vi "主程序.vi"() -> ()   [LabVIEW 2017, in "年前程序.lvlib"]
uses:
  <vilib>/Platform/TimedLoop/XDataNode/timing_clust.ctl
  <vilib>/Platform/TimedLoop/XDataNode/nitl_modes.ctl
  <vilib>/Platform/TimedLoop/XDataNode/wakeup.ctl
  <vilib>/myRIO/Common/Instrument Driver Framework/myRIO v1.0/UART/vis/myRIO v1.0 Close UART.vi
  <vilib>/FPGAPlugInAG/myRIO-1900/niLvFpga_Open_myRIO-1900.vi
  <vilib>/rvi/interface/common/dynamic/niFpgaDynamicAddResources.vi
  <vilib>/myRIO/Common/Instrument Driver Framework/Utilities/vis/FPGA Ref Manager.vi
  <vilib>/Utility/error.llb/Error Cluster From Error Code.vi
  <vilib>/myRIO/Common/Instrument Driver Framework/Utilities/vis/Ref Counter.vi
  <vilib>/FPGAPlugInAG/Dynamic/niLvFpga_Close_Dynamic.vi
  <vilib>/myRIO/Common/Instrument Driver Framework/myRIO v1.0/myRIO v1.0 Reset FPGA.vi
  <vilib>/myRIO/Common/Instrument Driver Framework/myRIO v1.0/IRQ/vis/myRIO v1.0 IRQ Info FGV.vi
  <vilib>/myRIO/Common/Instrument Driver Framework/myRIO v1.0/IRQ/vis/myRIO v1.0 Timer IRQ Info FGV.vi
  <vilib>/myRIO/Common/Instrument Driver Framework/myRIO v1.0/IRQ/vis/myRIO v1.0 ISR Agent.vi
  <vilib>/rvi/interface/nirviOpenFPGA/nirviOpenFPGA.xnode
  <vilib>/Platform/TimedLoop/XDataNode/XDataNode.xnode
  <vilib>/rvi/interface/nirviCloseFPGA/nirviCloseFPGA.xnode
  <vilib>/Platform/TimedLoop/XDataNode/XDNodeRunTimeDep.lvlib
  <vilib>/myRIO/Instrument Drivers/Utilities/Utilities.lvlib
panel:
  in  "最大速度":dbl
  in  "停止":bool
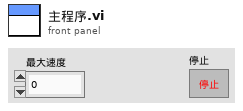
[diagram p1: front panel]
types:
  T1 = typedef "XDNodeRunTimeDep.lvlib/timing_clust.ctl" = cluster{"Expected End [f-1]":u64, "Actual End [f-1]":u64, "Finished Late? [f-1]":bool, "Expected End [i-1]":u64, "Actual End [i-1]":u64, "Finished Late? [i-1]":bool, "Expected Start [i]":u64, "Actual Start [i]":u64, "Expected Start [f]":u64, "Actual Start [f]":u64, "Source Name":string, "Structure Name":string, "Period":i64, "Deadline":i64, "Offset":i64, "Start":i64, "Priority":i32, "Timeout":i32, "Mode":T2, "Wakeup Reason":T3, "Error":errorcluster, "Source Type":string, "Secondary Source Type":string, "Global End Time":u64, "Global Start Time":u64, "Frame Duration":u64, "Iteration Duration":u64, "Assigned CPU":i32, "I/O Scan Engine Mode":u32}
  T2 = typedef "XDNodeRunTimeDep.lvlib/nitl_modes.ctl" = enum32{"No Change", "Process missed periods, maintain original phase", "Discard missed periods, maintain original phase", "Process missed periods, ignore original phase", "Discard missed periods, ignore original phase"}
  T3 = typedef "XDNodeRunTimeDep.lvlib/wakeup.ctl" = enum32{"Normal", "Aborted", "Asynchronous wakeup", "Timing source error", "Timed loop error", "Timeout"}
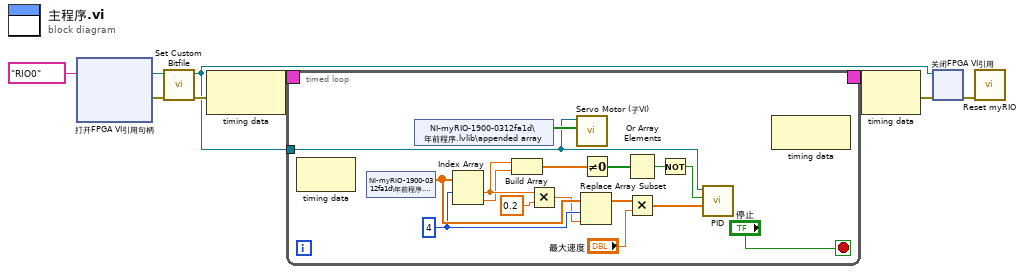
[diagram p0: block diagram]
diagram:
  n1 = xnode "打开FPGA VI引用句柄"("资源名称"=tag "RIO0") -> ("FPGA VI引用输出"=w5:refnum<k20>, "错误输出"=w4:errorcluster)  [unwired: 1 in]
  n2 = call <vilib>:"Set Custom Bitfile.vi"("error in (no error)"=w4, "Custom FPGA Reference In"=w5) -> ("error out"=w2:errorcluster, "Custom FPGA Reference Out"=w1:refnum<k20>)  [unwired: 8 in]
  n3 = node-c288(w2) -> (w9:T1)
  n4 = timed-loop {
    timing: w9 -> [_]
    timing-out: [_] -> w8
    tunnel: w1 -> [w21]
    stop <- "停止" stop-if-true
    w18 = 4 ("索引")
    n5 = node-c288() -> ()  [unwired: 1 in, 1 out]
    n6 = shared-variable "NI-myRIO-1900-0312fa1d\\年前程序.lvlib\\数组"() -> (w20:dbl[])  [unwired: 1 in, 1 out]
    n7 = shared-variable "NI-myRIO-1900-0312fa1d\\年前程序.lvlib\\appended array"() -> (w22:bool[])  [unwired: 1 in, 1 out]
    n8 = Index Array(array=w20, index #1=w18) -> (element #1=w15:dbl, element #2=w14:dbl)  [unwired: 1 in]
    n9 = Build Array(w15, w14) -> (w13:dbl[])
    n10 = Multiply(x=w15, y=0.2 ("x")) -> (x*y=w17:dbl)
    n11 = call "Servo Motor (子VI).vi"("Direction"=w22, "Custom FPGA Reference Out"=w21) -> ()  [unwired: 10 in]
    n12 = Replace Array Subset(array=w20, new element=w17, index=w18) -> (w19:dbl[])
    n13 = Not Equal To 0?(x=w13) -> (x != 0?=w12:bool[])
    n14 = Or Array Elements(Boolean array=w12) -> (logical OR=w11:bool)
    n15 = Multiply(x=w19, y="最大速度") -> (x*y=w23:dbl[])
    n16 = Not(x=w11) -> (.not. x?=w10:bool)
    n17 = call "PID.vi"("setpoint"=w23, "Relay"=w10, "Custom FPGA Reference Out"=w21) -> ()  [unwired: 9 in]
    n18 = node-c288() -> ()  [unwired: 1 in, 1 out]
  }
  n19 = node-c288(w8) -> (w7:errorcluster)
  n20 = xnode "关闭FPGA VI引用"("FPGA VI引用输入"=w1, "错误输入"=w7) -> ("错误输出"=w6:errorcluster)
  n21 = call <vilib>:"Reset myRIO.vi"("error in (no error)"=w6) -> ()  [unwired: 10 in, 1 out]
